vi "Show UI For Selection.vi"(8 "Error In":errorcluster, 11 "Pane Relief Main UI in":refnum<class "Pane Relief Main UI.lvclass">) -> (0 "Error Out":errorcluster, 3 "Pane Relief Main UI out":refnum<class "Pane Relief Main UI.lvclass">)   [LabVIEW 2018, in "Pane Relief Main UI.lvlib" / "Pane Relief Main UI.lvclass"]
uses:
  <resource>/dialog/QuickDrop/plugins/PaneRelief/Classes/Pane Relief Main UI/Pane Relief Main UI/Pane Relief Main UI.lvclass
  <resource>/dialog/QuickDrop/plugins/PaneRelief/Classes/Pane Relief Main UI/Pane Relief Main UI/Pane Relief Main UI.lvclass/Pane Relief Main UI.ctl
  <resource>/dialog/QuickDrop/plugins/PaneRelief/Classes/Panel Object/Panel Object.lvclass
  <vilib>/MGI/Panel Manager/Panel Actor/Panel Actor Messages/Show Panel Msg/Show Panel Msg.lvclass
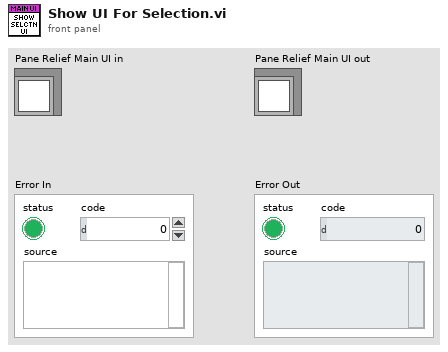
[diagram p1: front panel]
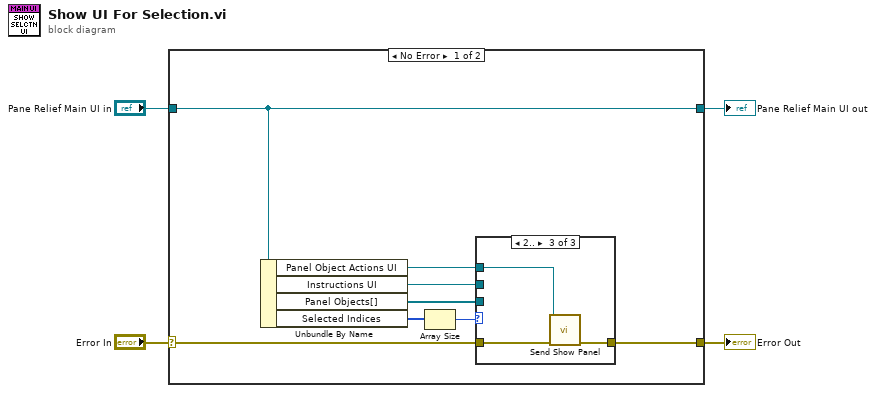
[diagram p0: block diagram]
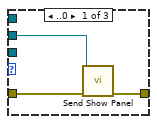
[diagram p2: hidden frame]
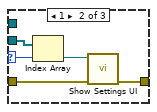
[diagram p3: hidden frame]
diagram:
  n1 = case shown="No Error" "Error In" {
    selector: "Error In" -> [w10 w25]
    tunnel: [w9 w25] -> w1
    tunnel: [w11 w24] -> w3
    tunnel: "Pane Relief Main UI in" -> [w11 w24]
    frame No Error {
      n2 = Unbundle By Name(w11) -> ("Panel Object Actions UI"=w5:refnum<class "Message Enqueuer.lvclass">, "Instructions UI"=w6:refnum<class "Message Enqueuer.lvclass">, "Panel Objects[]"=w12:refnum<class "Panel Object.lvclass">[], "Selected Indices"=w8:i32[])
      n3 = Array Size(array=w8) -> (size(s)=w7:i32)
      n4 = case shown="2.." w7 {
        selector: w7 -> [_ w16 _]
        tunnel: w12 -> [_ w20 _]
        tunnel: w10 -> [w14 w18 w22]
        tunnel: [w15 w17 w23] -> w9
        tunnel: w6 -> [w13 _ _]
        tunnel: w5 -> [_ _ w21]
        frame ..0 {
          n5 = call <vilib>:"Send Show Panel.vi"("Error In"=w14, "Message Enqueuer in"=w13) -> ("Error Out"=w15:errorcluster)  [unwired: 8 in, 1 out]
        }
        frame 1 {
          n6 = Index Array(array=w20, index=w16) -> (element=w19:refnum<class "Panel Object.lvclass">)
          n7 = call-dynamic "Show Settings UI.vi"("Error In"=w18, "Panel Object in"=w19) -> ("Error Out"=w17:errorcluster)  [unwired: 8 in, 1 out]
        }
        frame 2.. {
          n8 = call <vilib>:"Send Show Panel.vi"("Error In"=w22, "Message Enqueuer in"=w21) -> ("Error Out"=w23:errorcluster)  [unwired: 8 in, 1 out]
        }
      }
    }
    frame Error {
    }
  }
  "Pane Relief Main UI out" <- w3
  "Error Out" <- w1
